vi "Initialize Actor.vi"(7 "Host Name":string, 8 "error in (no error)":errorcluster, 9 "Actor Name":string, 10 "Message Broker Interface":refnum<class "Message Broker Interface.lvclass">, 11 "Terminal Timeout in":refnum<class "Terminal Timeout.lvclass">) -> (0 "error out":errorcluster, 3 "Terminal Timeout out":refnum<class "Terminal Timeout.lvclass">)   [LabVIEW 2016, in "CLD Exam - ATM.lvlib" / "Terminal Timeout.lvclass"]
uses:
  Terminal Timeout.lvclass
  Mediator/Classes/Message Broker Interface/Message Broker Interface.lvclass
  Terminal Timeout.lvclass/Terminal Timeout.ctl
  Mediator/Classes/Message Transport Event/Message Transport Event.lvclass
  D:/Repos/Stream/software/Mediator/Classes/Message Transport Interface/Message Transport Interface.lvclass
  Mediator/Classes/Mediated Synchronous Actor/Mediated Synchronous Actor.lvclass
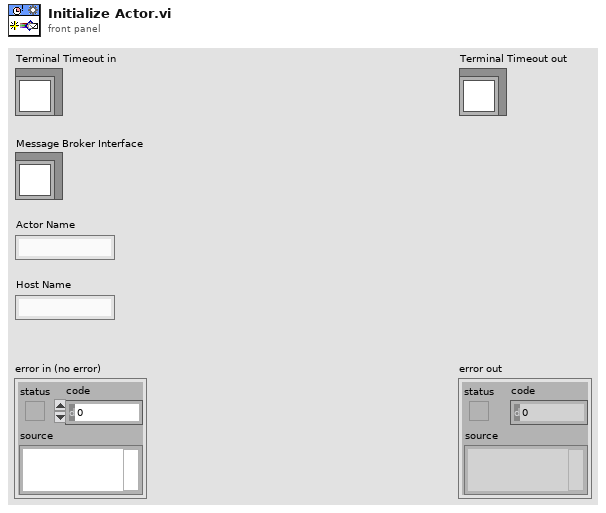
[diagram p1: front panel]
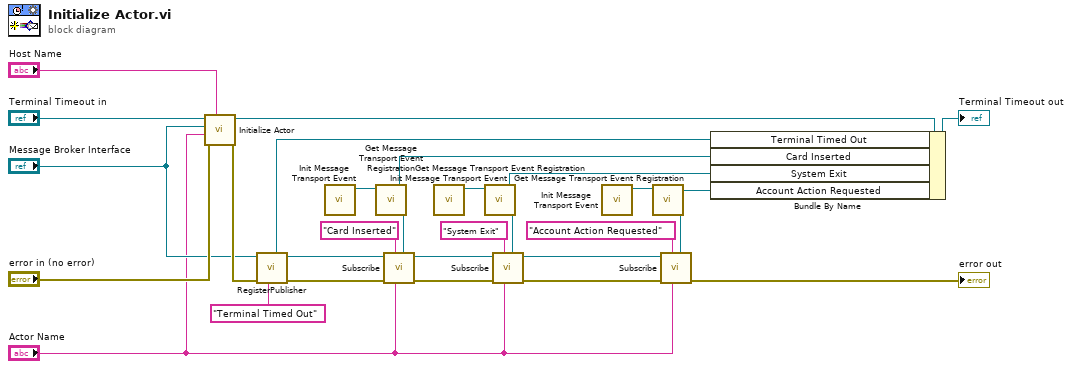
[diagram p0: block diagram]
diagram:
  n1 = call-parent "Initialize Actor.vi"("Host Name"="Host Name", "error in (no error)"="error in (no error)", "Actor Name"="Actor Name", "Message Broker Interface"="Message Broker Interface", "Mediated Synchronous Actor in"="Terminal Timeout in") -> ("error out"=w23:errorcluster, "Mediated Synchronous Actor out"=w26:refnum<class "Terminal Timeout.lvclass">)  [unwired: 5 in]
  n2 = call-dynamic "RegisterPublisher.vi"("Topic Name"="Terminal Timed Out", "error in (no error)"=w23, "Message Broker Interface in"="Message Broker Interface") -> ("error out"=w1:errorcluster, "Message Broker Interface out"=w2:refnum<class "Message Broker Interface.lvclass">, "Transport"=w21:refnum<class "Message Transport Queue.lvclass">)  [unwired: 4 in, 2 out]
  n3 = call "Init Message Transport Event.vi"() -> ("Message Transport Event out"=w18:refnum<class "Message Transport Event.lvclass">)  [unwired: 10 in, 1 out]
  n4 = call "Get Message Transport Event Registration.vi"("Message Transport Event in"=w18) -> ("Event Registration Refnum"=w12:refnum<event-registration>, "Message Transport Event out"=w19:refnum<class "Message Transport Event.lvclass">)  [unwired: 7 in, 2 out]
  n5 = call-dynamic "Subscribe.vi"("Message Transport Interface"=w19, "Subscriber Name"="Actor Name", "Topic Name"="Card Inserted", "error in (no error)"=w1, "Message Broker Interface in"=w2) -> ("error out"=w13:errorcluster, "Message Broker Interface out"=w14:refnum<class "Message Broker Interface.lvclass">)  [unwired: 4 in, 1 out]
  n6 = call "Init Message Transport Event.vi"() -> ("Message Transport Event out"=w17:refnum<class "Message Transport Event.lvclass">)  [unwired: 10 in, 1 out]
  n7 = call "Get Message Transport Event Registration.vi"("Message Transport Event in"=w17) -> ("Event Registration Refnum"=w11:refnum<event-registration>, "Message Transport Event out"=w16:refnum<class "Message Transport Event.lvclass">)  [unwired: 7 in, 2 out]
  n8 = call-dynamic "Subscribe.vi"("Message Transport Interface"=w16, "Subscriber Name"="Actor Name", "Topic Name"="System Exit", "error in (no error)"=w13, "Message Broker Interface in"=w14) -> ("error out"=w7:errorcluster, "Message Broker Interface out"=w6:refnum<class "Message Broker Interface.lvclass">)  [unwired: 4 in, 1 out]
  n9 = call "Init Message Transport Event.vi"() -> ("Message Transport Event out"=w8:refnum<class "Message Transport Event.lvclass">)  [unwired: 10 in, 1 out]
  n10 = call "Get Message Transport Event Registration.vi"("Message Transport Event in"=w8) -> ("Event Registration Refnum"=w4:refnum<event-registration>, "Message Transport Event out"=w9:refnum<class "Message Transport Event.lvclass">)  [unwired: 7 in, 2 out]
  n11 = call-dynamic "Subscribe.vi"("Message Transport Interface"=w9, "Subscriber Name"="Actor Name", "Topic Name"="Account Action Requested", "error in (no error)"=w7, "Message Broker Interface in"=w6) -> ("error out"=→"error out":errorcluster)  [unwired: 4 in, 2 out]
  n12 = Bundle By Name(cluster=w26, "Terminal Timed Out"=w21, "Card Inserted"=w12, "System Exit"=w11, "Account Action Requested"=w4) -> (→"Terminal Timeout out":refnum<class "Terminal Timeout.lvclass">)
